vi "State Machine.vi"   [LabVIEW 2020]
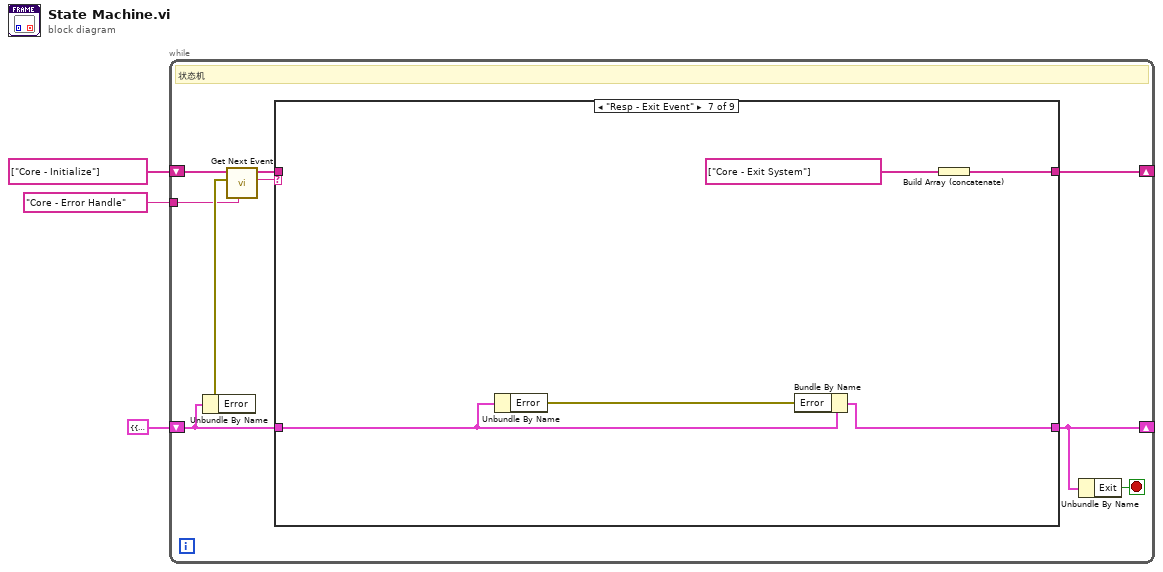
[diagram p0: block diagram]
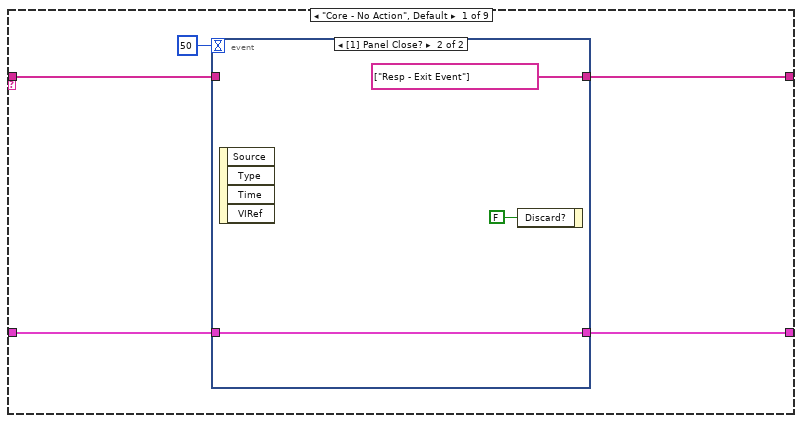
[diagram p2: hidden frame]
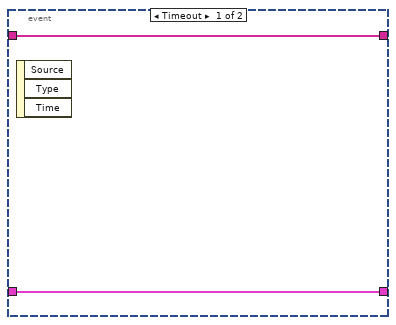
[diagram p3: hidden frame]
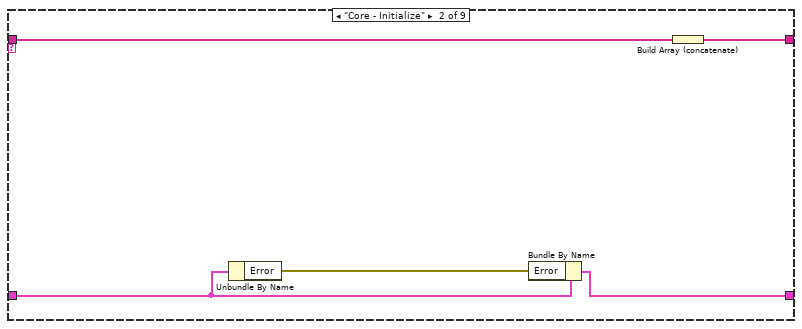
[diagram p4: hidden frame]
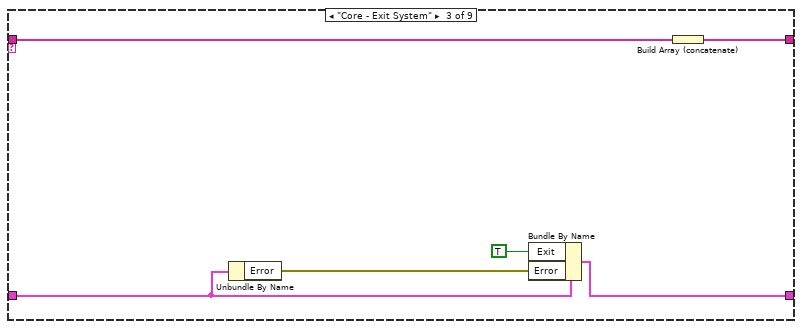
[diagram p5: hidden frame]
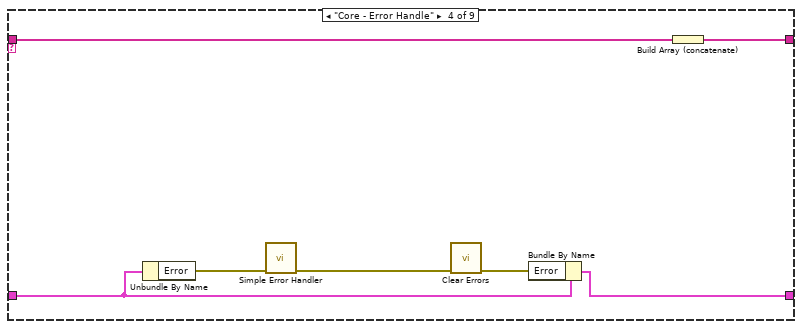
[diagram p6: hidden frame]
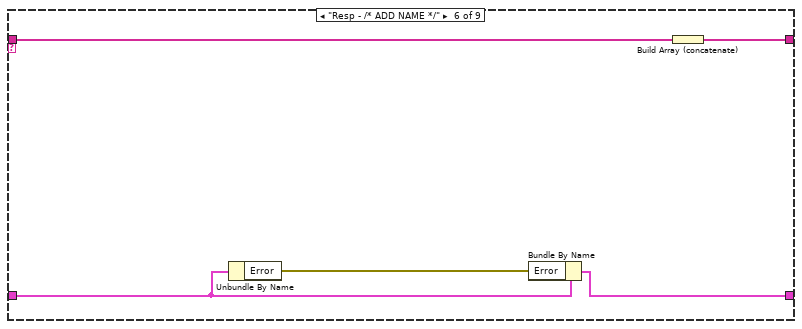
[diagram p8: hidden frame]
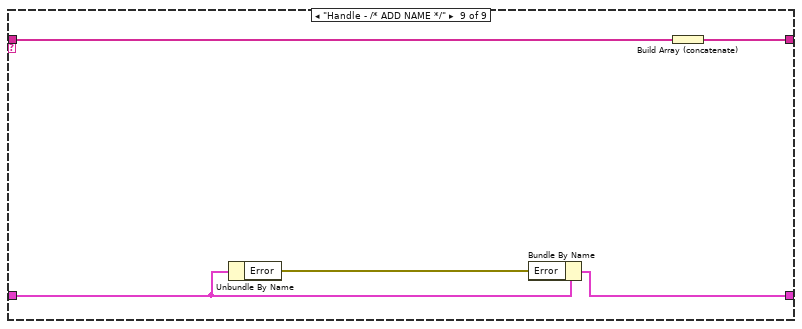
[diagram p10: hidden frame]
diagram:
  n1 = while {
    shift-right: [w7] -> _
    shift-left: string[] ["Core - Initialize"] -> [w10]
    shift-right: [w6] -> _
    shift-left: cluster{"Error":errorcluster, "Exit":bool} {"Error"={"status"=FALSE, "code"=0, "source"=""}, "Exit"=FALSE} ("Temp Variable") -> [w9]
    tunnel: "Core - Error Handle" ("Error Handle") -> [w4]
    stop <- w5 stop-if-true
    # "状态机"
    n2 = Unbundle By Name(w9) -> ("Error"=w8:errorcluster)
    n3 = call "Get Next Event.vi"("Error Handle"=w4, "error in (no error)"=w8, "event queue in"=w10) -> ("next event"=w11:string, "event queue out"=w12:string[])  [unwired: 7 in]
    n4 = case shown="\"Resp - Exit Event\"" w11 {
      tunnel: w12 -> [w14 w27 w33 w40 w42 w47 _ w53 w59]
      tunnel: w9 -> [w16 w25 w31 w38 w41 w45 w51 w54 w57]
      tunnel: [w13 w26 w32 w39 w42 w46 w52 w53 w58] -> w7
      tunnel: [w15 w23 w30 w37 w41 w44 w50 w54 w56] -> w6
      frame "Core - No Action", Default {
        n5 = event shown="[1] Panel Close?" {
          selector: _ -> [_ _]
          dyn-events: _ -> [_ _]
          timeout: 50 -> [_ _]
          tunnel: w16 -> [w19 w22]
          tunnel: [w19 w22] -> w15
          tunnel: w14 -> [w18 _]
          tunnel: [w18 string[] ["Resp - Exit Event"] ("event queue out")] -> w13
          event Timeout {
            n6 = event-data() -> ()  [unwired: 1 in, 3 out]
          }
          event Panel Close? {
            n7 = event-data() -> ()  [unwired: 1 in, 4 out]
            n8 = event-data("Discard?"=FALSE) -> ()  [unwired: 1 in, 1 out]
          }
        }
      }
      frame "Core - Initialize" {
        n9 = Unbundle By Name(w25) -> ("Error"=w24:errorcluster)
        n10 = Bundle By Name(cluster=w25, "Error"=w24) -> (w23:cluster{"Error":errorcluster, "Exit":bool})
        n11 = Build Array (concatenate)(w27) -> (w26:string[])
      }
      frame "Core - Exit System" {
        n12 = Unbundle By Name(w31) -> ("Error"=w29:errorcluster)
        n13 = Bundle By Name(cluster=w31, "Exit"=TRUE, "Error"=w29) -> (w30:cluster{"Error":errorcluster, "Exit":bool})
        n14 = Build Array (concatenate)(w33) -> (w32:string[])
      }
      frame "Core - Error Handle" {
        n15 = Unbundle By Name(w38) -> ("Error"=w36:errorcluster)
        n16 = call <vilib>:"Simple Error Handler.vi"("error in (no error)"=w36) -> ("error out"=w34:errorcluster)  [unwired: 4 in, 4 out]
        n17 = call <vilib>:"Clear Errors.vi"("error in (no error)"=w34) -> ("error out"=w35:errorcluster)  [unwired: 5 in, 1 out]
        n18 = Bundle By Name(cluster=w38, "Error"=w35) -> (w37:cluster{"Error":errorcluster, "Exit":bool})
        n19 = Build Array (concatenate)(w40) -> (w39:string[])
      }
      frame "---------------------------------Response---------------------------------" {
      }
      frame "Resp - /* ADD NAME */" {
        n20 = Unbundle By Name(w45) -> ("Error"=w43:errorcluster)
        n21 = Bundle By Name(cluster=w45, "Error"=w43) -> (w44:cluster{"Error":errorcluster, "Exit":bool})
        n22 = Build Array (concatenate)(w47) -> (w46:string[])
      }
      frame "Resp - Exit Event" {
        n23 = Unbundle By Name(w51) -> ("Error"=w49:errorcluster)
        n24 = Bundle By Name(cluster=w51, "Error"=w49) -> (w50:cluster{"Error":errorcluster, "Exit":bool})
        n25 = Build Array (concatenate)(string[] ["Core - Exit System"] ("event queue out")) -> (w52:string[])
      }
      frame "----------------------------------Execute-----------------------------------" {
      }
      frame "Handle - /* ADD NAME */" {
        n26 = Unbundle By Name(w57) -> ("Error"=w55:errorcluster)
        n27 = Bundle By Name(cluster=w57, "Error"=w55) -> (w56:cluster{"Error":errorcluster, "Exit":bool})
        n28 = Build Array (concatenate)(w59) -> (w58:string[])
      }
    }
    n29 = Unbundle By Name(w6) -> ("Exit"=w5:bool)
  }
